vi "Link Parameters.vi"(7 "Parameter W Table in":refnum<class "Registry.lvclass">, 8 "error in (no error)":errorcluster, 10 "Parameter R Table in":refnum<class "Registry.lvclass">, 11 "Major Frame in":refnum<class "Major Frame.lvclass">) -> (0 "error out":errorcluster, 2 "Parameter R Table out":refnum<class "Registry.lvclass">, 5 "Parameter W Table out":refnum<class "Registry.lvclass">)   [LabVIEW 2020, in "BCI-1553 API.lvlib" / "Major Frame.lvclass"]
doc: "<DO NOT CALL>\n\nThis method is leveraged by the Bus Controller to properly link the Major Frame parameters.\n\nLinks tables to parameters and their data pointers."
uses:
  Major Frame.lvclass
  Dependencies/Registry/Registry.lvclass
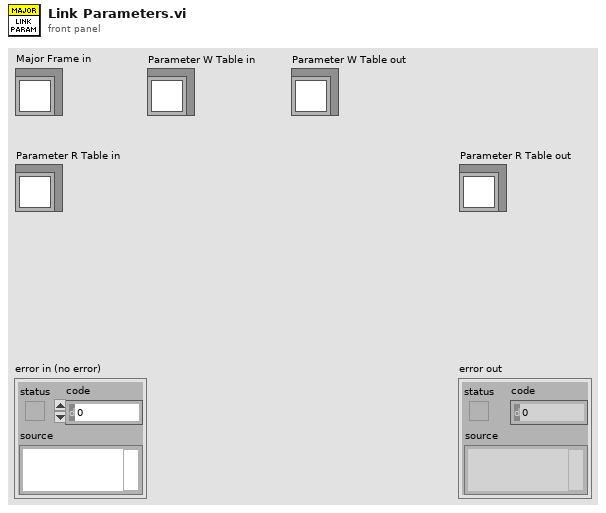
[diagram p1: front panel]
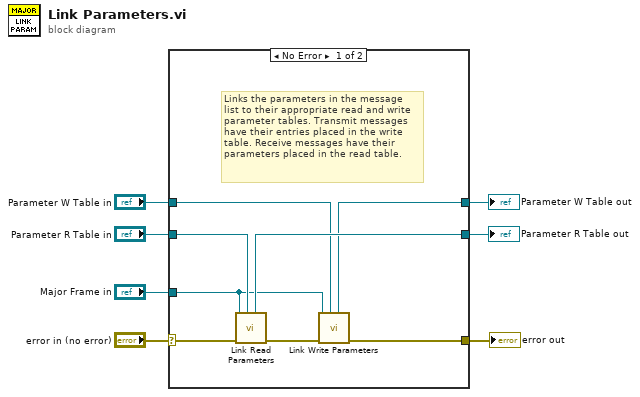
[diagram p0: block diagram]
diagram:
  n1 = case shown="No Error" "error in (no error)" {
    selector: "error in (no error)" -> [w9 w18]
    tunnel: [w8 w18] -> w6
    tunnel: "Major Frame in" -> [w13 _]
    tunnel: [w11 w17] -> w4
    tunnel: "Parameter W Table in" -> [w12 w17]
    tunnel: [w14 w16] -> w2
    tunnel: "Parameter R Table in" -> [w15 w16]
    frame No Error {
      # "Links the parameters in the message\nlist to their appropriate read and write\nparameter tables. Transmit messages\nhave their entries placed in the write\ntable. Receive messages have their\nparameters placed in the read table."
      n2 = call "Link Read Parameters.vi"("Parameter R Table in"=w15, "error in (no error)"=w9, "Major Frame in"=w13) -> ("error out"=w10:errorcluster, "Parameter R Table out"=w14:refnum<class "Registry.lvclass">)  [unwired: 7 in]
      n3 = call "Link Write Parameters.vi"("Parameter W Table in"=w12, "error in (no error)"=w10, "Major Frame in"=w13) -> ("error out"=w8:errorcluster, "Parameter W Table out"=w11:refnum<class "Registry.lvclass">)  [unwired: 7 in]
    }
    frame Error {
    }
  }
  "error out" <- w6
  "Parameter W Table out" <- w4
  "Parameter R Table out" <- w2
